vi "浮点数组转字符串数组.vi"(8 "小数点位数(默认3位)":i32=3, 10 "浮点数组":dbl[](array[numeric])) -> (2 "Str数组":string[](array[string]))   [LabVIEW 2014]
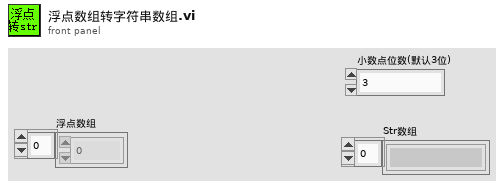
[diagram p1: front panel]
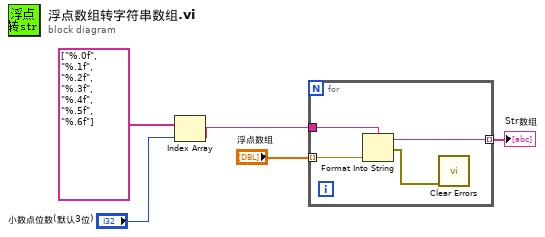
[diagram p0: block diagram]
diagram:
  n1 = Index Array(array=string[] ["%.0f", "%.1f", "%.2f", "%.3f", "%.4f", "%.5f", "%.6f"], index="小数点位数(默认3位)") -> (element=w1:string)
  n2 = for {
    tunnel: "浮点数组" -> [w9] mode=indexing
    tunnel: [w8] -> w5 mode=indexing
    tunnel: w1 -> [w6]
    n3 = Format Into String(format string=w6, w9) -> (resulting string=w8:string, error out=w7:errorcluster)  [unwired: 2 in]
    n4 = call <vilib>:"Clear Errors.vi"("error in (no error)"=w7) -> ()  [unwired: 5 in, 2 out]
  }
  "Str数组" <- w5
